vi "Lead Compensator.vi"() -> ()   [LabVIEW 2019]
uses:
  <vilib>/Simulation/Scripting/Companion Diagram/SimConfigNode/SimParams.ctl
  <vilib>/Simulation/Scripting/Companion Diagram/SimConfigNode/_simSolvers.ctl
  <vilib>/Simulation/Implementation/Shared/SIMSCR Execution Mode.ctl
  <vilib>/Platform/TimedLoop/XDataNode/timing_clust.ctl
  <vilib>/Platform/TimedLoop/XDataNode/nitl_modes.ctl
  <vilib>/Platform/TimedLoop/XDataNode/wakeup.ctl
  <vilib>/Simulation/Param Hierarchy/Typedefs/SIMPH Param Control Actions.ctl
  <vilib>/Simulation/Implementation/Shared/SIM limit type.ctl
  <vilib>/Simulation/Implementation/Shared/NILVSim_ParamChanged.vi
  <vilib>/Simulation/Implementation/Shared/NILVSim_FinishedLate.vi
  <vilib>/Simulation/Implementation/Shared/NILVSIM_BeginStep.vi
  <vilib>/Simulation/DataSources/Implementation/NILVSim Signal Generator.llb/SIM Signal Generator (scalar).vi
  <vilib>/Simulation/Utility/Implementation/SIM Halt.vi
  <vilib>/Simulation/ContinuousLinear/Implementation/NILVSim Transfer Function Direct.llb/SIM Transfer Function Direct (SISO).vi
  <vilib>/Simulation/SignalArithmetic/Implementation/NILVSim Gain.llb/SIM Gain (scalar).vi
  <vilib>/Simulation/SignalDisplay/Implementation/NILVSim Time Waveform.llb/SIM Time Waveform (vector).vi
  <vilib>/Simulation/ContinuousLinear/Implementation/NILVSim Integrator new.llb/SIM Integrator distributor (scalar).vi
  <vilib>/Simulation/ContinuousLinear/Implementation/NILVSim Integrator new.llb/SIM Integrator collector (scalar).vi
  <vilib>/Simulation/Nonlinear/Implementation/NILVSim Saturation.llb/SIM Saturation (scalar).vi
  <vilib>/Simulation/SignalDisplay/Implementation/NILVSim Time Waveform.llb/SIM Time Waveform (scalar).vi
  <vilib>/Simulation/Implementation/Shared/NILVSim_Manager.vi
  <vilib>/Utility/error.llb/Clear Errors.vi
  <vilib>/Simulation/Implementation/Shared/NILVSim_FinalizeModel.vi
  <vilib>/Simulation/Implementation/Shared/SIM Unbundle Sim Info.vi
  <vilib>/Simulation/Implementation/Shared/SIMSH Read Queue.vi
  <vilib>/Simulation/Implementation/Shared/NILVSim_Initialize.vi
  SubVIs/Encoders.vi
  <vilib>/Simulation/Utility/Implementation/NILVSim Get Time and IsAcceptedStep.vi
  SubVIs/Motor.vi
  <vilib>/Simulation/Implementation/Shared/NILVSim_GetModelError.vi
  <vilib>/Simulation/Implementation/Shared/SIM Bundle Sim Info.vi
  <vilib>/Simulation/Scripting/Companion Diagram/SimConfigNode/SimDog.xnode
  <vilib>/Platform/TimedLoop/XDataNode/XDataNode.xnode
  <vilib>/Simulation/Implementation/XNodeFramework/SimXNode/SimX.xnode
  <vilib>/Simulation/ContinuousLinear/Implementation/NILVSim Integrator new.llb/SIM Integrator (scalar).vi
  <vilib>/Platform/TimedLoop/XDataNode/XDNodeRunTimeDep.lvlib
  <vilib>/Simulation/Implementation/Shared/NI_SIM_Implementation.lvlib
panel:
  in  "K_c":dbl=1.0
  in  "Stop Button":bool
  in  "Signal Generator":T1={"Amplitude (rad/s)"=10.0, "Frequency (Hz)"=0.2, "Offset (rad/s)"=30.0} {"Frequency (Hz)" step=0.1}
  out "Motor Voltage":waveform(dbl)(graph)={"t0"=timestamp(19.19 s since 1904-01-01), "dt"=1.0, "Y"=[1.7574388110467847]}
  out "Motor Speed":waveform(dbl)[](graph)=[{"t0"=timestamp(19.19 s since 1904-01-01), "dt"=1.0, "Y"=[40.0]}, {"t0"=timestamp(19.19 s since 1904-01-01), "dt"=1.0, "Y"=[40.39795078767929]}]
  out "Error":errorcluster={"status"=FALSE, "code"=-363017, "source"="ELVIS III v1.0 Write PWM.vi"}
  # "Engineering Trainer Boards"
  # "Controls Board"
  # "Lead Compensator"
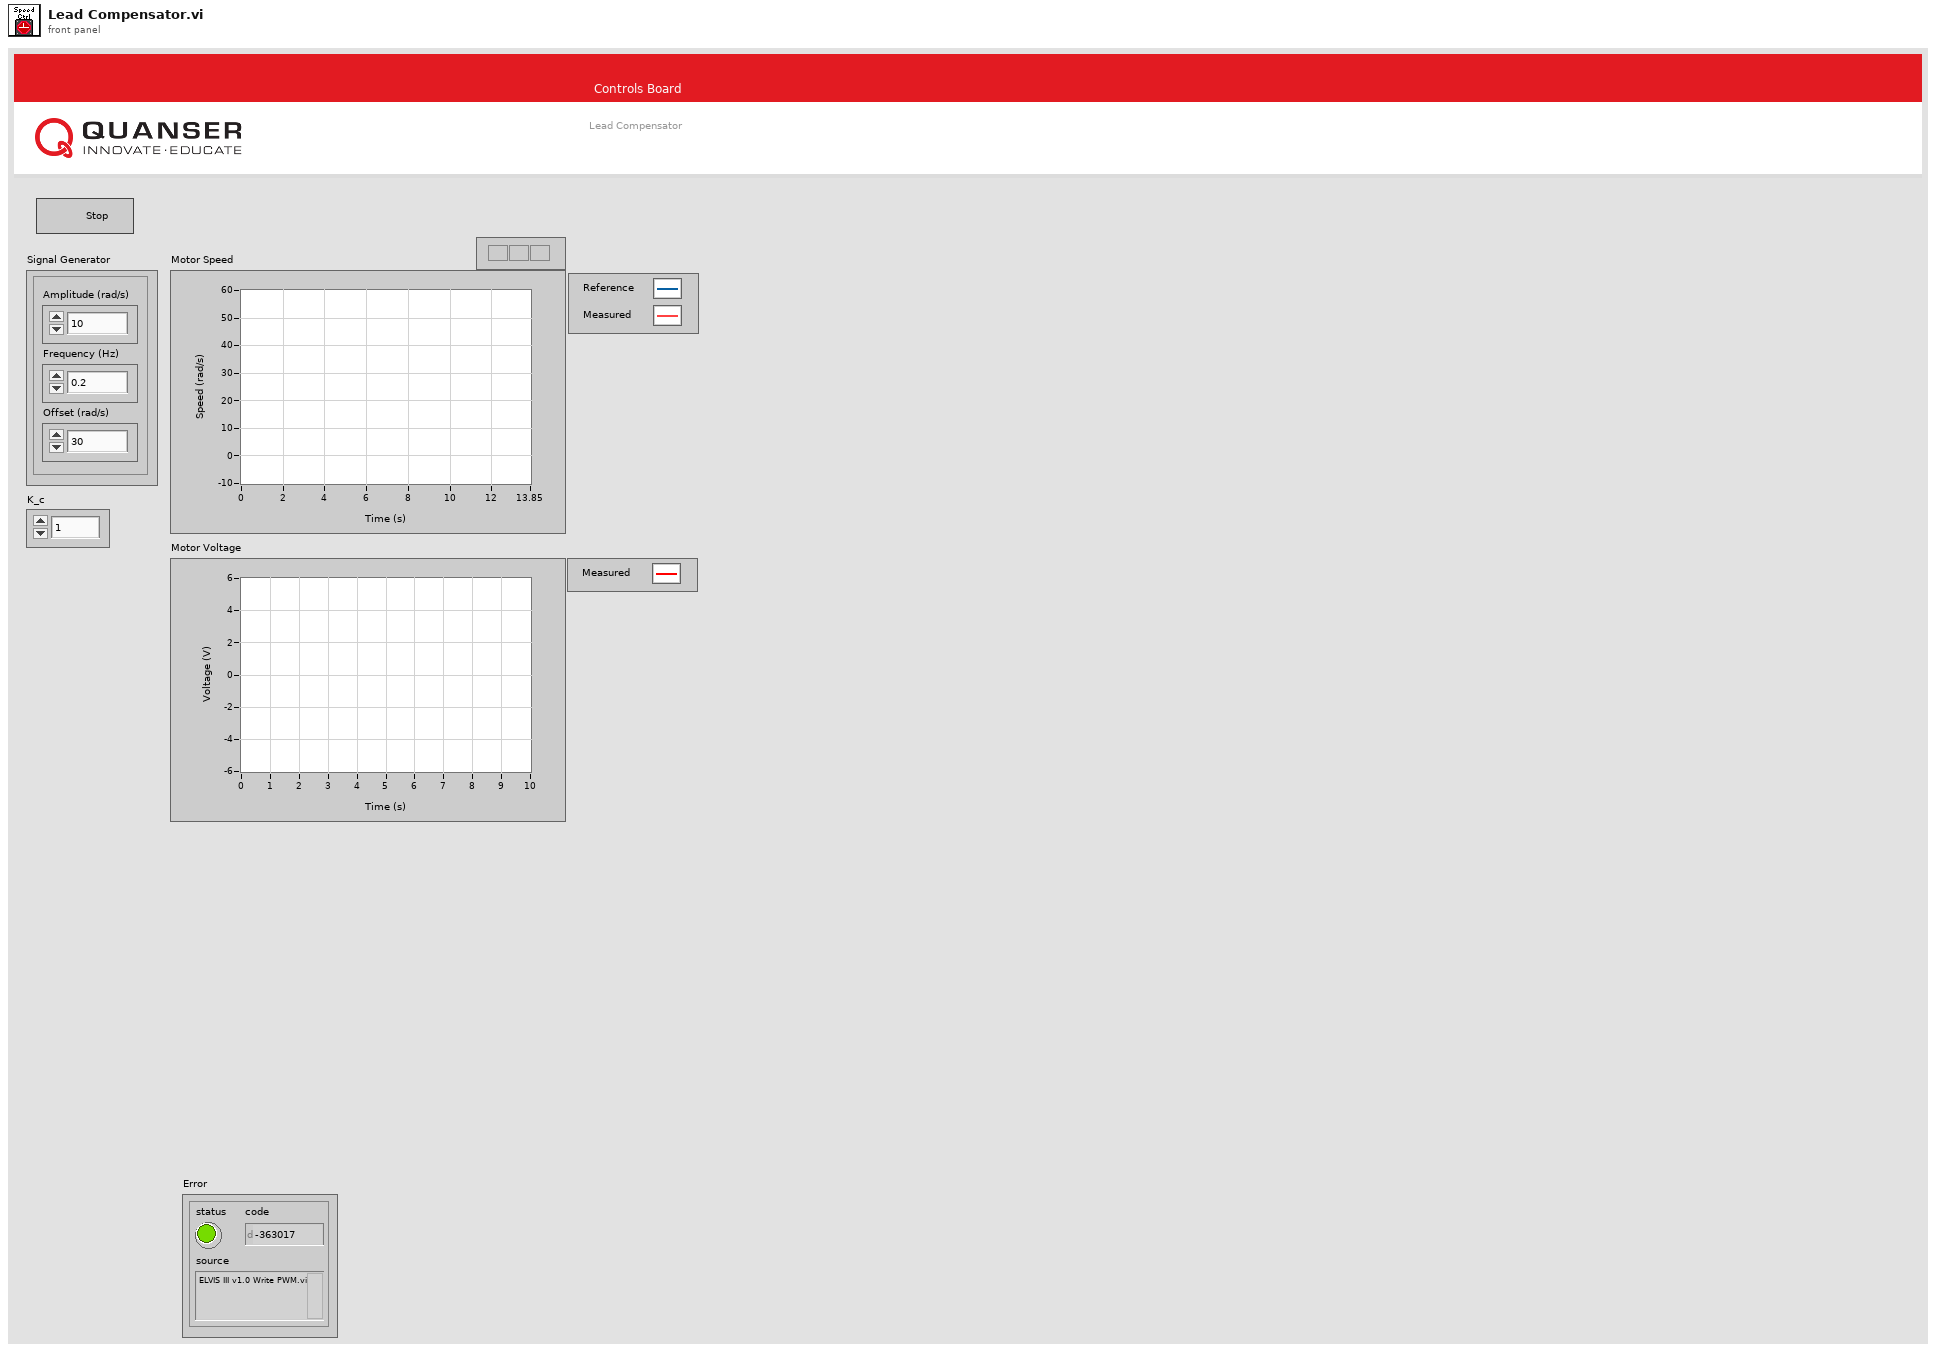
[diagram p1: front panel]
types:
  T1 = cluster{"Amplitude (rad/s)":dbl, "Frequency (Hz)":dbl, "Offset (rad/s)":dbl}
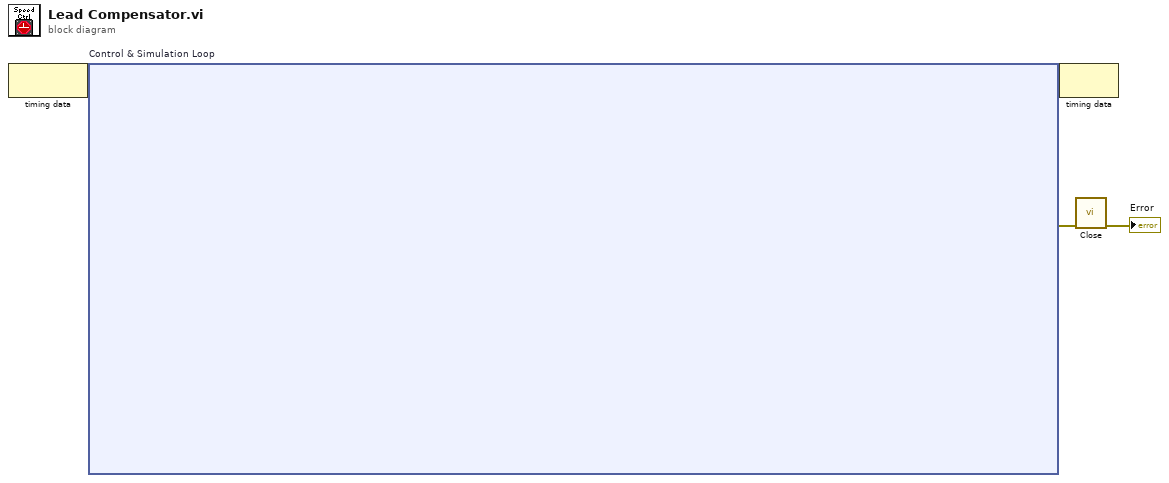
[diagram p0: block diagram]
diagram:
  n1 = node-c288() -> (w4:variant)  [unwired: 1 in]
  n2 = node-c254 "Control & Simulation Loop"(w4) -> (w3:variant, w2:errorcluster)
  n3 = node-c288(w3) -> ()  [unwired: 1 out]
  n4 = call "Close.vi"("error in"=w2) -> ("error out"=→"Error":errorcluster)  [unwired: 10 in]
